vi "Write File.vi"(8 "error in (no error)":errorcluster, 10 "File":path, 11 "TDMS Properties in":refnum<class "TDMS Properties.lvclass">) -> (0 "error out":errorcluster, 3 "TDMS Properties out":refnum<class "TDMS Properties.lvclass">)   [LabVIEW 2019, in "TDMS Properties.lvclass"]
uses:
  TDMS Properties.lvclass
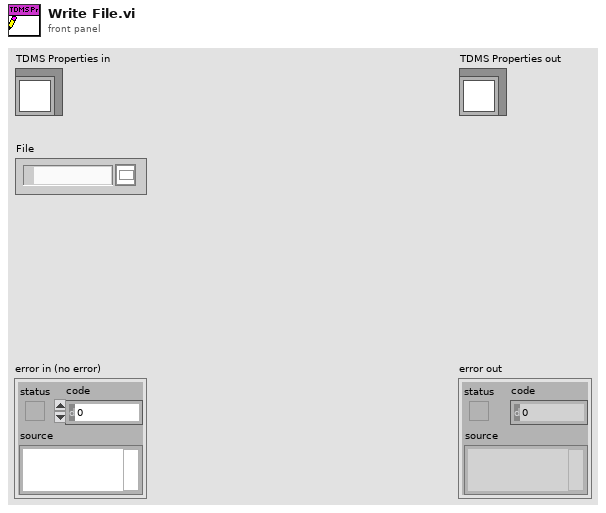
[diagram p1: front panel]
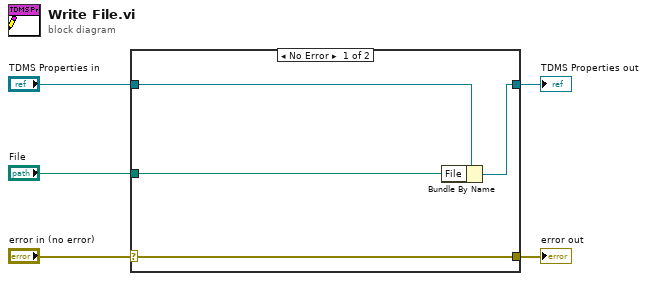
[diagram p0: block diagram]
diagram:
  n1 = case shown="No Error" "error in (no error)" {
    selector: "error in (no error)" -> [w9 w10]
    tunnel: [w9 w10] -> w4
    tunnel: [w7 w11] -> w2
    tunnel: "TDMS Properties in" -> [w8 w11]
    tunnel: "File" -> [w6 _]
    frame No Error {
      n2 = Bundle By Name(cluster=w8, "File"=w6) -> (w7:refnum<class "TDMS Properties.lvclass">)
    }
    frame Error {
    }
  }
  "error out" <- w4
  "TDMS Properties out" <- w2
